vi "关闭照明灯.vi"(8 "error in (no error)":errorcluster caption="错误输入（无错误）", 11 "钻床基本操作 输入":refnum<class "钻床基本操作.lvclass"> caption="DNL_LabVIEW Object in") -> (0 "error out":errorcluster caption="错误输出", 3 "钻床基本操作 输出":refnum<class "钻床基本操作.lvclass"> caption="DNL_LabVIEW Object out")   [LabVIEW 2011, in "钻床基本操作.lvclass"]
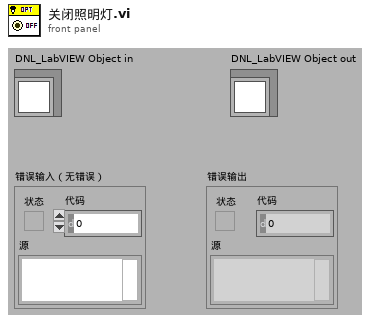
[diagram p1: front panel]
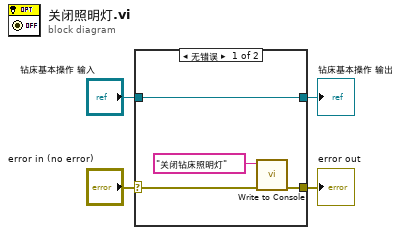
[diagram p0: block diagram]
diagram:
  n1 = case shown="无错误" "error in (no error)" {
    selector: "error in (no error)" -> [w7 w10]
    tunnel: [w6 w10] -> w3
    tunnel: [w8 w9] -> w1
    tunnel: "钻床基本操作 输入" -> [w8 w9]
    frame No Error {
      n2 = call "Write to Console.vi"("error in (no error)"=w7, "Input"="关闭钻床照明灯") -> ("error out"=w6:errorcluster)  [unwired: 9 in]
    }
    frame Error {
    }
  }
  "error out" <- w3
  "钻床基本操作 输出" <- w1
